vi "Synchronous Latch.vi"(9 "clear":bool=TRUE, 10 "set":bool=TRUE) -> (2 "out":bool=TRUE)   [LabVIEW 2020]
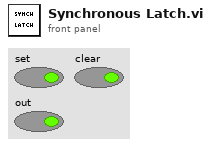
[diagram p1: front panel]
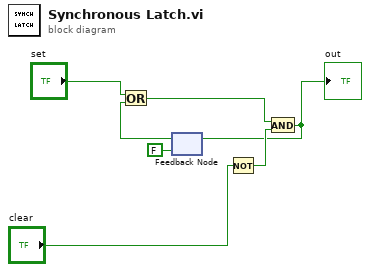
[diagram p0: block diagram]
diagram:
  n1 = feedback #1(FALSE) -> (w6:bool)
  n2 = Or(x="set", y=w6) -> (x .or. y?=w5:bool)
  n3 = Not(x="clear") -> (.not. x?=w4:bool)
  n4 = And(x=w5, y=w4) -> (x .and. y?=w1:bool)
  "out" <- w1
  n5 = feedback-in #1(w1) -> ()
